vi "Convert Old data to new format.vi"   [LabVIEW 2017]
types:
  T1 = enum16{"open", "open or create", "create or replace", "create", "open (read only)"}
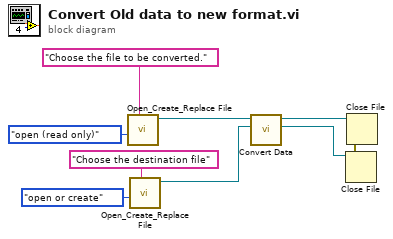
[diagram p0: block diagram]
diagram:
  n1 = call <vilib>:"Open_Create_Replace File.vi"("prompt"="Choose the file to be converted.", "function (open:0)"=T1."open (read only)") -> ("refnum"=w9:refnum<file>)  [unwired: 6 in, 3 out]
  n2 = call <vilib>:"Open_Create_Replace File.vi"("prompt"="Choose the destination file", "function (open:0)"=T1."open or create") -> ("refnum"=w3:refnum<file>)  [unwired: 6 in, 3 out]
  n3 = call <vilib>:"Convert Data.vi"("refnum to write"=w3, "refnum to read"=w9) -> ("refnum to write 2"=w5:refnum<file>, "refnum to read 2"=w7:refnum<file>)  [unwired: 7 in, 1 out]
  n4 = Close File(refnum=w5) -> (error out=w6:errorcluster)  [unwired: 1 in, 1 out]
  n5 = Close File(refnum=w7, error in=w6) -> ()  [unwired: 2 out]
